vi "FTW-Consumer-Construct.vi"(5 "Address":string, 11 "error in":errorcluster) -> (4 "FTW-Consumer Out":refnum<class "FTW-Consumer.lvclass">, 6 "Actual Address":string, 10 "Event Registration Refnum":refnum<event-registration>, 15 "error out":errorcluster)   [LabVIEW 2013, in "FTW-Consumer.lvclass"]
uses:
  FTW-Consumer.lvclass
  Package/Base/FTW-Message.lvclass
  Ether/FTW-Ether-EndpointType.ctl
  Endpoint/FTW-Endpoint.lvclass
  FTW-Consumer.lvclass/FTW-Consumer.ctl
  FTW-Consumer-Worker.vi
  Ether/FTW-Ether.lvclass
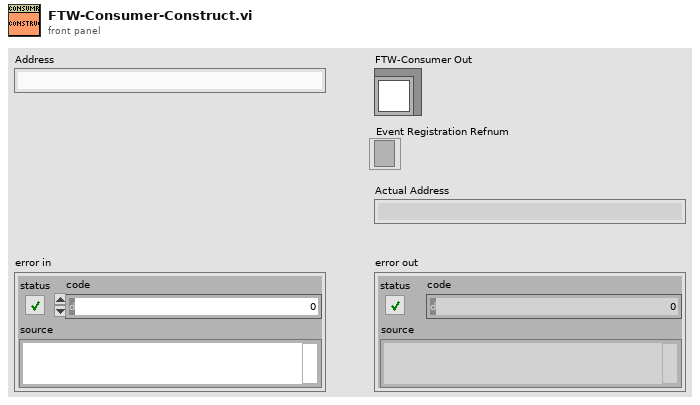
[diagram p1: front panel]
types:
  T1 = typedef "FTW-Ether.lvclass/FTW-Ether-EndpointType.ctl" = enum16{"Server", "Client", "Publisher", "Subscriber"}
  T2 = typedef "FTW-Ether.lvclass/FTW-Ether-MessageTransportScheme.ctl" = enum16{"In process (inproc://)", "TCP (tcp://)"}
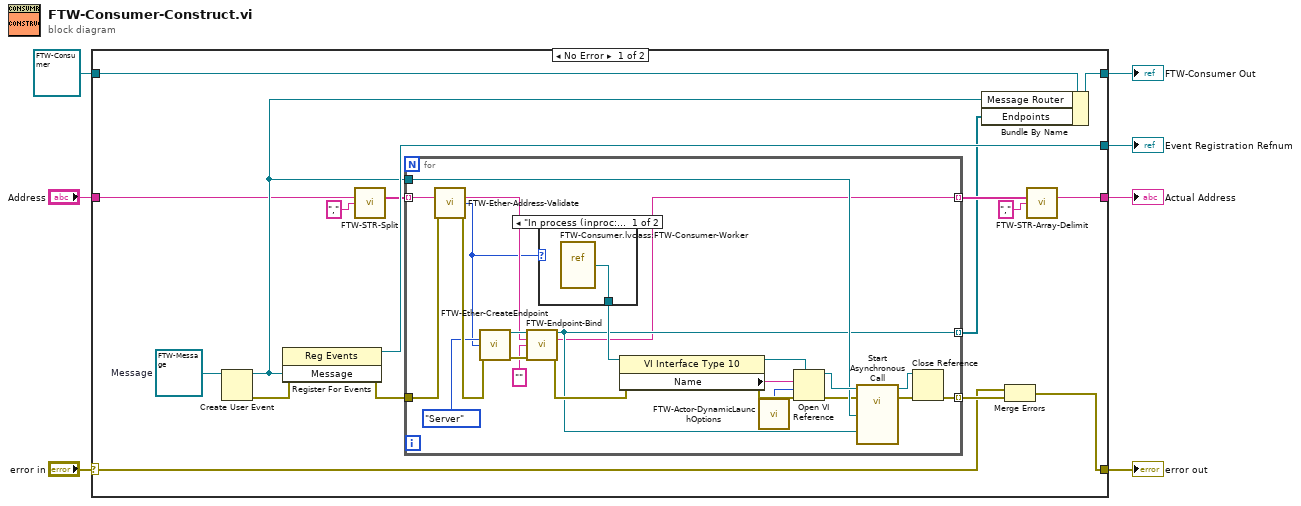
[diagram p0: block diagram]
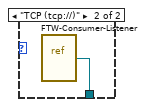
[diagram p2: hidden frame]
diagram:
  n1 = case shown="No Error" "error in" {
    selector: "error in" -> [w9 w51]
    tunnel: [w11 w51] -> w6
    tunnel: [w24 w50] -> w5
    tunnel: [w23 _] -> w1
    tunnel: "Address" -> [w15 _]
    tunnel: [w13 _] -> w3
    tunnel: refnum<class "FTW-Consumer.lvclass"> refnum ("LVmsg_Router.lvclass") -> [w19 w50]
    frame No Error {
      w22 = refnum<class "FTW-Message.lvclass"> refnum  # Message
      n2 = Create User Event(user event datatype=w22) -> (user event=w20:refnum<user-event>, error out=w17:errorcluster)  [unwired: 1 in]
      n3 = register-events(error in=w17, w20) -> (reference out=w23:refnum<event-registration>, error out=w10:errorcluster)  [unwired: 1 in]
      n4 = call "FTW-STR-Split.vi"("Delimited String"=w15, "Delimiter"=",") -> ("Array of Strings"=w8:string[])  [unwired: 13 in]
      n5 = for {
        tunnel: [w25] -> w21 mode=indexing
        tunnel: w20 -> [w35]
        tunnel: w10 -> [w33]
        tunnel: [w31] -> w18 mode=indexing
        tunnel: w8 -> [w30] mode=indexing
        tunnel: [w29] -> w14 mode=indexing
        n6 = call "FTW-Ether-Address-Validate.vi"("Address"=w30, "error in"=w33) -> ("Sanitized Address"=w36:string, "Message Transport Scheme"=w27:T2, "error out"=w37:errorcluster)  [unwired: 11 in]
        n7 = call "FTW-Ether-CreateEndpoint.vi"("Endpoint Type"=FTW-Ether-EndpointType."Server", "Message Transport Scheme"=w27, "error in"=w37) -> ("FTW Endpoint"=w39:refnum<class "FTW-Endpoint.lvclass">, "error out"=w38:errorcluster)  [unwired: 11 in]
        n8 = call-dynamic "FTW-Endpoint-Bind.vi"("FTW Endpoint"=w39, "Endpoint Address"=w36, "Requested Identity"="", "error in"=w38) -> ("FTW Endpoint out"=w29:refnum<class "FTW-Endpoint.lvclass">, "Actual Endpoint Address"=w25:string, "error out"=w34:errorcluster)  [unwired: 8 in, 1 out]
        n9 = case shown="\"In process (inproc://)\"" w27 {
          tunnel: [w48 w49] -> w47
          frame "In process (inproc://)" {
            n10 = vi-ref "FTW-Consumer.lvclass:FTW-Consumer-Worker.vi"() -> (w48:refnum<vi>)
          }
          frame "TCP (tcp://)" {
            n11 = vi-ref "FTW-Consumer-Listener.vi"() -> (w49:refnum<vi>)
          }
        }
        n12 = property class="VI Interface Type 10"(reference=w47, error in=w34) -> (reference out=w43:refnum<vi>, error out=w46:errorcluster, "Name"=w45:string)
        n13 = call "FTW-Actor-DynamicLaunchOptions.vi"() -> ("Open VI Ref Options"=w44:i32)
        n14 = Open VI Reference(type specifier VI Refnum (for type only)=w43, vi path=w45, options=w44, error in (no error)=w46) -> (vi reference=w41:refnum<vi>, error out=w32:errorcluster)  [unwired: 2 in]
        n15 = call-by-ref "Start Asynchronous Call"(reference=w41, error in=w32, "Endpoint"=w29, "Message Handler"=w35) -> (reference out=w40:refnum<vi>, error out=w42:errorcluster)  [unwired: 1 in]
        n16 = Close Reference(reference=w40, error in (no error)=w42) -> (error out=w31:errorcluster)
      }
      n17 = Bundle By Name(cluster=w19, "Message Router"=w20, "Endpoints"=w14) -> (w24:refnum<class "FTW-Consumer.lvclass">)
      n18 = Merge Errors(w9, w18) -> (w11:errorcluster)
      n19 = call "FTW-STR-Array-Delimit.vi"("Array of Strings"=w21, "Delimiter"=",") -> ("Delimited String"=w13:string)  [unwired: 13 in]
    }
    frame Error {
    }
  }
  "FTW-Consumer Out" <- w5
  "error out" <- w6
  "Actual Address" <- w3
  "Event Registration Refnum" <- w1
